vi "project.vi"() -> ()   [LabVIEW 2021]
uses:
  <vilib>/MakerHub/LINX/Public/Peripherals/Digital/Digital Read 1 Chan.vi
  <vilib>/MakerHub/LINX/Public/Peripherals/Digital/Digital Write 1 Chan.vi
  <vilib>/MakerHub/LINX/Public/Peripherals/Digital/Digital Read N Chans.vi
  <vilib>/MakerHub/LINX/Public/Peripherals/Digital/Digital Write N Chans.vi
  <vilib>/MakerHub/LINX/Private/Local IO/LinxDigitalRead.vi
  <vilib>/MakerHub/LINX/Public/Utilities/Check Channel.vi
  <vilib>/MakerHub/LINX/Private/Local IO/LinxDigitalWrite.vi
  <vilib>/MakerHub/LINX/Public/Utilities/Open Serial.vi
  <vilib>/MakerHub/LINX/Public/Sensors/Motion/Servo/Servo Open One Channel.vi
  <vilib>/MakerHub/LINX/Public/Sensors/Motion/Servo/Servo Set Pulse Width One Channel.vi
  <vilib>/MakerHub/LINX/Private/Utilties/Generate Error.vi
  <vilib>/MakerHub/LINX/Public/Sensors/Motion/Servo/Servo Close One Channel.vi
  <vilib>/MakerHub/LINX/LMH-LINX.lvlib
  <vilib>/MakerHub/LINX/Public/Sensors/Distance/Ultrasonic/Ultrasonic.lvlib
  <vilib>/MakerHub/LINX/Public/Sensors/Motion/Servo/Servo.lvlib
panel:
  in  "Servo Channel":u8
  in  "Serial Port":refnum<visa-resource-name>="N/A"
  in  "Servo Motor Controller":dbl(knob) scale=500.0..2500.0
  out "Alarm":bool
  out "Meters":dbl(knob) scale=0.02..20.0
  in  "stop":bool
  # "Distance Sensor"
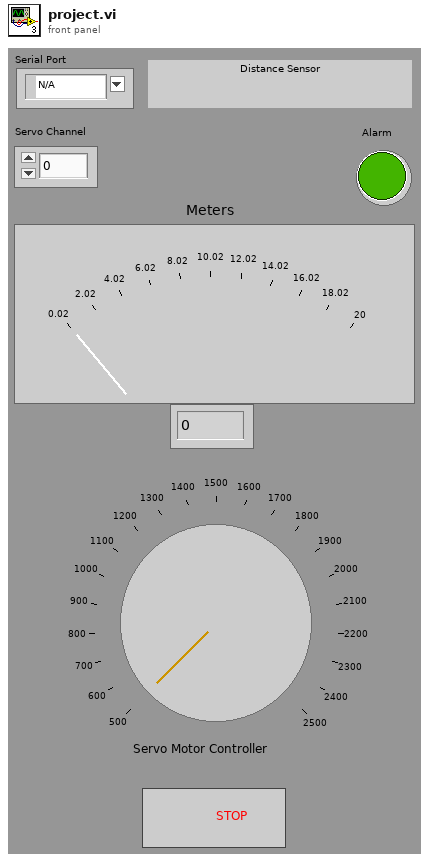
[diagram p1: front panel]
types:
  T1 = typedef "LMH-LINX.lvlib/LINX Ref.ctl" = cluster{"IO":T2, "Interface":T3, "LINX Device Config":T4}
  T2 = typedef "LMH-LINX.lvlib/Platform.ctl" = enum16{"Remote", "Local"}
  T3 = typedef "LMH-LINX.lvlib/Interface.ctl" = enum16{"Serial", "TCP"}
  T4 = typedef "LMH-LINX.lvlib/Device.lvlib/LINX Device Config.ctl" = cluster{"Interface":T3, "COM Port":refnum<visa-resource-name>, "TCP Configuration":T5, "Device Family":u8, "Device ID":u8, "Device Name":string, "TCP Ref":refnum<k5>, "Channels":T6}
  T5 = typedef "LMH-LINX.lvlib/Device.lvlib/TCP Config.ctl" = cluster{"IP Address":string, "Port":u16}
  T6 = typedef "LMH-LINX.lvlib/Channels.ctl" = cluster{"DI":u8[], "DO":u8[], "AI":u8[], "AO":u8[], "PWM":u8[], "QE":u8[], "UART":u8[], "I2C 2":u8[], "SPI":u8[], "CAN":u8[], "Servo":u8[], "AI Ref (V)":dbl, "AI Resolution (Bits)":u8, "AO Ref (V)":dbl, "AO Resolution (Bits)":u8}
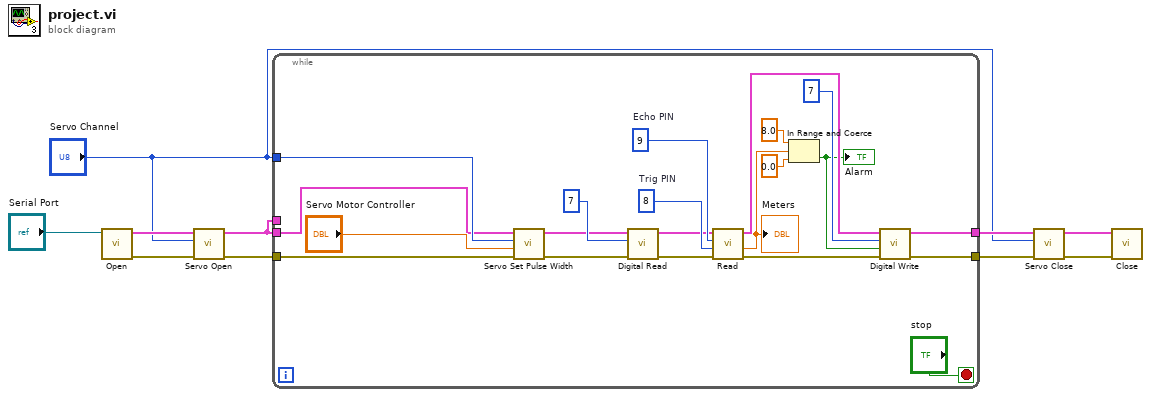
[diagram p0: block diagram]
diagram:
  n1 = call-poly <vilib>:"Open.vi"("Serial Port"="Serial Port") -> ("Error Out"=w9:errorcluster, "LINX Resource"=w10:T1)  [unwired: 8 in, 1 out]
  n2 = call-poly <vilib>:"Servo Open.vi"("Error In"=w9, "Servo Channel"="Servo Channel", "LINX Resource"=w10) -> ("Error Out"=w1:errorcluster, "LINX Resource"=w2:T1)  [unwired: 7 in]
  n3 = while {
    tunnel: w2 -> [_]
    tunnel: [w16] -> w7
    tunnel: [w15] -> w5
    tunnel: "Servo Channel" -> [w14]
    tunnel: w2 -> [w11]
    tunnel: w1 -> [w12]
    stop <- "stop" stop-if-true
    w29 = u8 8  # Trig PIN
    w30 = u8 9  # Echo PIN
    n4 = call-poly <vilib>:"Servo Set Pulse Width.vi"("Error In"=w12, "Pulse Width (uS)"="Servo Motor Controller", "Servo Channel"=w14, "LINX Resource"=w11) -> ("Error Out"=w17:errorcluster, "LINX Resource"=w18:T1)  [unwired: 6 in]
    n5 = call-poly <vilib>:"Digital Read.vi"("Error In"=w17, "DI Channel"=u8 7, "LINX Resource"=w18) -> ("Error Out"=w27:errorcluster, "LINX Resource"=w28:T1)  [unwired: 6 in, 1 out]
    n6 = call <vilib>:"Read.vi"("Error In"=w27, "DO Channel"=w29, "DI Channel"=w30, "LINX Resource"=w28) -> ("Error Out"=w23:errorcluster, "Centimeters"=w24:dbl, "LINX Resource"=w22:T1)  [unwired: 4 in, 1 out]
    "Meters" <- w24
    n7 = In Range and Coerce(upper limit=8.0, x=w24, lower limit=0.0) -> (In Range?=w19:bool)  [unwired: 1 out]
    "Alarm" <- w19
    n8 = call-poly <vilib>:"Digital Write.vi"("Error In"=w23, "Output Value"=w19, "DO Channel"=u8 7, "LINX Resource"=w22) -> ("Error Out"=w15:errorcluster, "LINX Resource"=w16:T1)  [unwired: 6 in]
  }
  n9 = call-poly <vilib>:"Servo Close.vi"("Error In"=w5, "Servo Channel"="Servo Channel", "LINX Resource"=w7) -> ("Error Out"=w6:errorcluster, "LINX Resource"=w8:T1)  [unwired: 7 in]
  n10 = call <vilib>:"Close.vi"("Error In"=w6, "LINX Resource"=w8) -> ()  [unwired: 9 in, 1 out]
